vi "CreateNewStringWithSubstitute.vi"(0 "Subject":string, 1 "CompileOptions":u32 format="%.0x", 2 "pCompileContext":u64 format="%.0x", 5 "search pattern":string, 7 "Replacement":string, 9 "Offset":u64, 11 "error in":errorcluster, 12 "MatchOptions":u32 format="%.0x", 13 "pMatchContext":u64 format="%.0x") -> (4 "OutString":string, 15 "error out":errorcluster)   [LabVIEW 2021, in "libpcre2-8.lvlib"]
uses:
  libpcre2-8.lvlib
  Pcre2CompileError.vi
  Pcre2ErrorNull.vi
  Pcre2LibError.vi
  Pcre2FnkCallError.vi
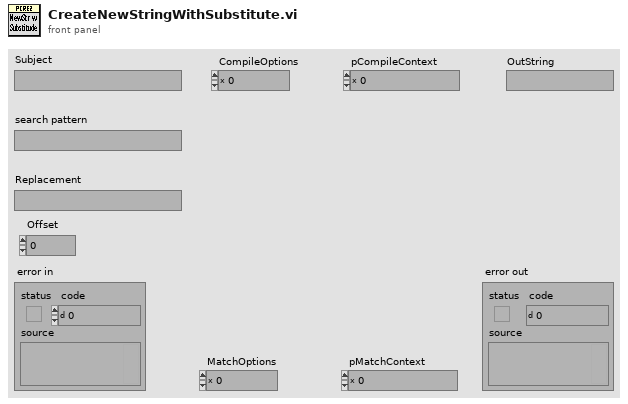
[diagram p1: front panel]
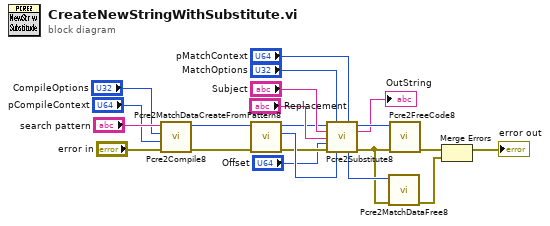
[diagram p0: block diagram]
diagram:
  n1 = call "Pcre2Compile8.vi"("error in"="error in", "pCompileContext"="pCompileContext", "Options"="CompileOptions", "Pattern"="search pattern") -> ("error out"=w20:errorcluster, "pCode"=w19:u64)  [unwired: 6 in]
  n2 = call "Pcre2MatchDataCreateFromPattern8.vi"("error in"=w20, "pCode"=w19) -> ("error out"=w13:errorcluster, "pMatchData"=w14:u64, "pCode"=w7:u64)  [unwired: 7 in]
  n3 = call "Pcre2Substitute8.vi"("pCode"=w7, "Options"="MatchOptions", "pMatchContext"="pMatchContext", "Subject"="Subject", "Replacement"="Replacement", "StartOffset"="Offset", "error in"=w13, "pMatchData"=w14) -> ("pCode"=w8:u64, "OutString"=→"OutString":string, "pMatchData"=w9:u64, "error out"=w5:errorcluster)  [unwired: 4 in]
  n4 = call "Pcre2MatchDataFree8.vi"("error in"=w5, "pMatchData"=w9) -> ("error out"=w2:errorcluster)  [unwired: 9 in]
  n5 = call "Pcre2FreeCode8.vi"("error in"=w5, "pCode"=w8) -> ("error out"=w3:errorcluster)  [unwired: 9 in]
  n6 = Merge Errors(w3, w2) -> (→"error out":errorcluster)
